vi "Write Harmonics.vi"(8 "error in (no error)":errorcluster, 10 "Harmonics":i8[](array[numeric]), 11 "Harmonics in":refnum<class "Harmonics.lvclass">) -> (0 "error out":errorcluster, 3 "Harmonics out":refnum<class "Harmonics.lvclass">)   [LabVIEW 2016, in "Harmonics.lvlib" / "Harmonics.lvclass"]
uses:
  Harmonics.lvclass
  Harmonics.lvclass/Harmonics.ctl
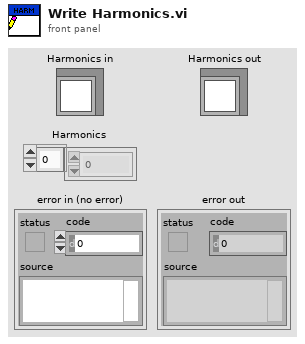
[diagram p1: front panel]
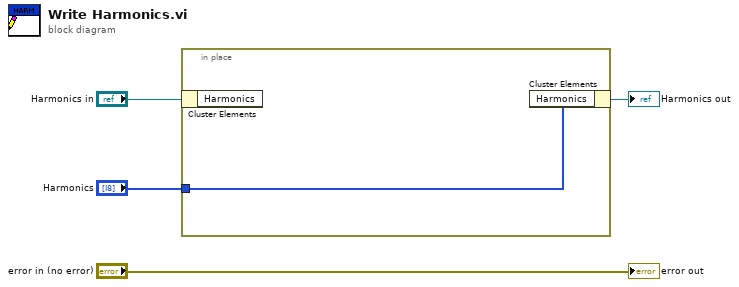
[diagram p0: block diagram]
diagram:
  n1 = in-place {
    in-place-border: "Harmonics" -> [w5]
    n2 = in-place-cluster #1("Harmonics in") -> ()  [unwired: 1 out]
    n3 = in-place-cluster #1("Harmonics"=w5) -> (→"Harmonics out":refnum<class "Harmonics.lvclass">)
  }
  "error out" <- "error in (no error)"
